vi "UDP_WR.vi"(1 "DATA":u32 format="%x", 2 "ADDRESS":u16) -> (0 "REG_WR":string)   [LabVIEW 2016]
doc: "This VI is designed to be used with the UDP Receiver VI. Run the UDP Receiver.vi first.\n\nThe UDP protocol differs from TCP in that there is no error-checking with the packets of information that are sent, and thus no guarantee whatsoever that an intended recipient will actually receive a given piece of data.\n\nUDP does offer the ability to \"broadcast\" data across a network--simply specify an IP Address of all ones (255.255.255.255) to attempt to broadcast information network-wide. Keep in mind that routers and other network hardware will generally refuse to forward the broadcast beyond certain points, so the extent of the broadcast will in practice be limited."
uses:
  D:/share/SBND/SBND_SW/SBND_WIB_DLL/WIB_DLL/bin/Debug/WIB_DLL.dll
  SBND/SBND_SW/SBND_WIB_DLL/WIB_DLL/bin/Debug/WIB_DLL.dll
  WIB_Global.vi
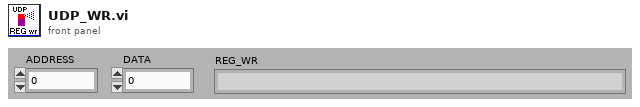
[diagram p1: front panel]
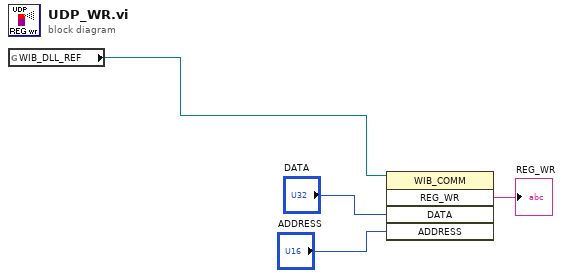
[diagram p0: block diagram]
diagram:
  n1 = global read "WIB_Global.vi" "WIB_DLL_REF"() -> (w1:refnum<k24>)
  n2 = invoke class="WIB_COMM" method="REG_WR"(reference=w1, "DATA"="DATA", "ADDRESS"="ADDRESS") -> ("REG_WR"=→"REG_WR":string)  [unwired: 2 in, 4 out]
